vi "9-1.vi"() -> (3 "Numeric":i32)   [LabVIEW 2022 SP3, in "AoC22.lvlib"]
uses:
  AoC22.lvlib
  <vilib>/Utility/miscctls.llb/LVMapReplaceAction.ctl
  <vilib>/IlluminatedG/lv-stream/Stream.lvlib
panel:
  in  "OK Button":bool
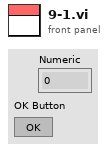
[diagram p1: front panel]
types:
  T1 = map{cluster{"Row":i32, "Col":i32}, cluster{"Tail Count":i32}}
  T2 = typedef "LVMapReplaceAction.ctl" = enum32{"Modify Entry only if found", "Add or Modify Entry", "Delete Entry"}
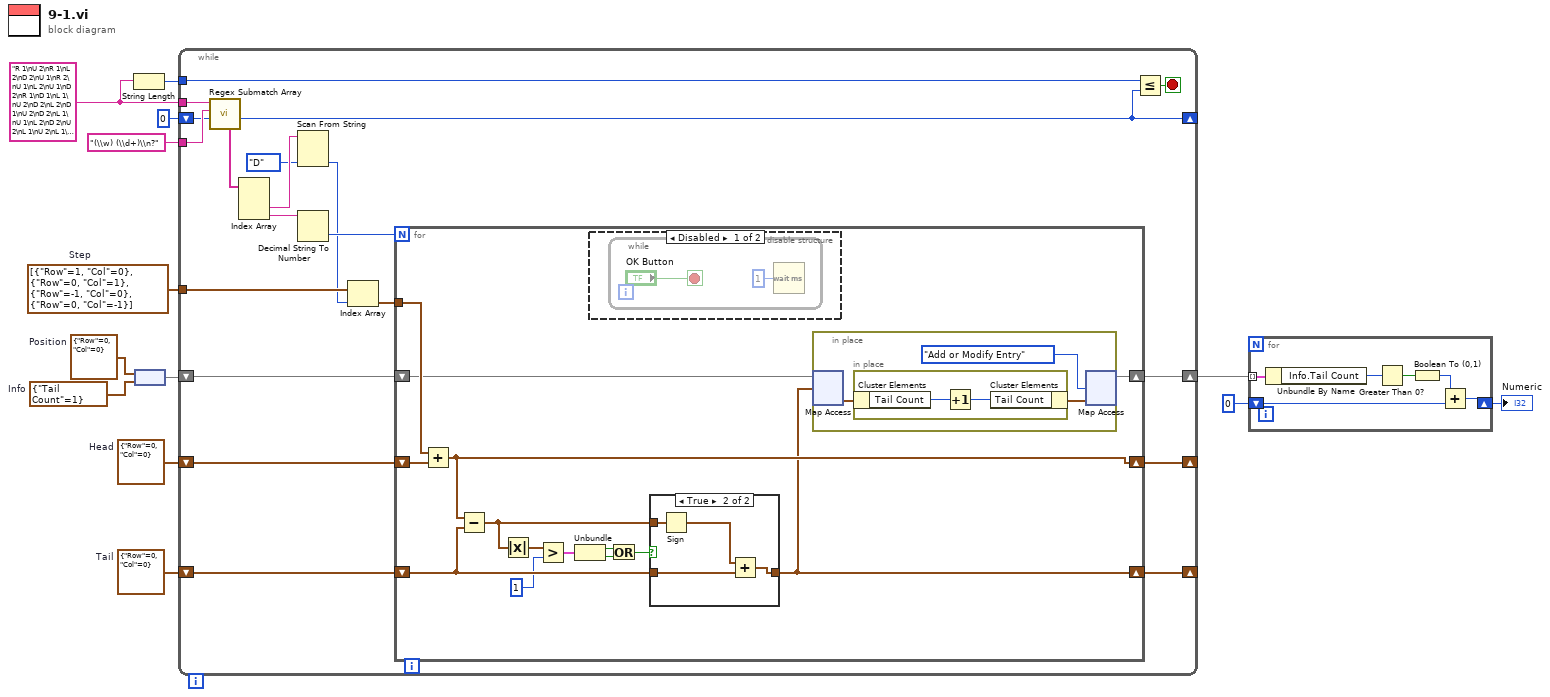
[diagram p0: block diagram]
diagram:
  w4 = cluster{"Tail Count":i32} {"Tail Count"=1}  # Info
  w6 = cluster{"Row":i32, "Col":i32} {"Row"=0, "Col"=0}  # Position
  w7 = cluster{"Row":i32, "Col":i32}[] [{"Row"=1, "Col"=0}, {"Row"=0, "Col"=1}, {"Row"=-1, "Col"=0}, {"Row"=0, "Col"=-1}]  # Step
  w11 = cluster{"Row":i32, "Col":i32} {"Row"=0, "Col"=0}  # Tail
  w12 = cluster{"Row":i32, "Col":i32} {"Row"=0, "Col"=0}  # Head
  w9 = "R 1\nU 2\nR 1\nL 2\nD 2\nU 1\nR 2\nU 1\nL 2\nU 1\nD 2\nR 1\nD 1\nL 1\nU 2\nD 2\nL 2\nD 1\nU 2\nD 2\nL 1\nU 1\nL 2\nD 2\nU 2\nL 1\nU 2\nL 1\nR 2\nU 1\nL 1\nR 2\nD 1\nU 2\nR 1\nU 1\nR 2\nU 1\nR 2\nU 1\nD 1\nU 1\nD 1\nL 2\nD 2\nR 1\nU 1\nR 1\nU 1\nL 1\nU 1\nD 2\nR 2\nD 2\nL 2\nU 2\nR 1\nD 1\nU 1\nD 2\nR 1\nD 2\nL 2\nR 2\nL 1\nU 1\nL 2\nD 2\nL 2\nD 1\nR 1\nL 2\nD 2\nR 1\nL 1\nR 1\nD 1\nR 1\nD 2\nL 2\nU 1\nD 2\nR 2\nD 1\nU 1\nL 1\nD 1\nU 2\nR 1\nU 1\nL 2\nU 1\nL 1\nU 2\nL 2\nD 2\nU 1\nL 1\nU 2\nD 2\nL 2\nD 2\nR 2\nU 2\nL 2\nD 1\nU 1\nR 2\nD 2\nL 2\nR 2\nD 2\nL 1\nD 1\nU 2\nR 2\nD 3\nR 1\nU 3\nL 3\nD 2\nR 1\nD 1\nL 2\nD 1\nR 2\nU 3\nL 2\nU 2\nR 3\nU 3\nL 1\nD 3\nR 3\nU 2\nR 3\nU 3\nL 1\nD 3\nR 3\nL 2\nR 2\nL 3\nD 3\nR 2\nD 2\nR 2\nD 1\nR 1\nL 1\nD 2\nR 1\nD 2\nU 1\nR 2\nL 2\nR 2\nU 2\nR 2\nD 1\nU 1\nD 1\nL 3\nU 3\nD 3\nL 1\nU 2\nR 2\nU 2\nR 1\nU 1\nL 2\nU 2\nR 3\nU 1\nD 3\nR 3\nU 2\nR 1\nU 1\nD 3\nL 2\nU 3\nL 1\nR 2\nD 3\nR 2\nU 1\nR 2\nD 1\nU 3\nL 2\nD 1\nR 1\nL 3\nR 3\nD 2\nR 1\nU 2\nR 3\nD 2\nU 2\nL 2\nU 1\nR 2\nU 2\nL 2\nD 3\nL 2\nD 1\nL 1\nU 2\nL 1\nD 2\nR 1\nD 2\nR 1\nL 2\nU 1\nL 1\nU 1\nD 2\nR 4\nD 4\nL 2\nR 4\nD 1\nL 2\nD 2\nL 4\nU 4\nD 4\nL 3\nR 3\nD 1\nL 1\nD 1\nU 4\nR 4\nU 4\nD 2\nR 1\nU 3\nR 2\nU 3\nR 4\nD 3\nU 3\nL 4\nD 1\nR 2\nU 3\nD 4\nU 3\nR 2\nL 1\nD 2\nU 2\nR 3\nU 2\nR 2\nD 2\nL 2\nU 4\nR 1\nL 3\nR 1\nL 1\nD 3\nR 4\nD 2\nR 4\nU 3\nL 1\nD 1\nR 4\nU 3\nD 1\nL 3\nR 1\nL 3\nD 2\nL 2\nR 3\nL 4\nD 4\nU 1\nL 1\nR 1\nD 3\nL 2\nR 1\nD 3\nR 2\nD 4\nU 4\nR 3\nU 1\nD 3\nL 3\nD 3\nU 1\nD 2\nU 4\nR 4\nU 2\nD 1\nR 1\nD 4\nL 2\nR 3\nU 4\nL 1\nD 1\nU 4\nL 3\nD 4\nU 2\nR 4\nU 2\nR 4\nU 2\nL 1\nR 1\nL 3\nD 4\nL 2\nR 2\nL 3\nU 3\nR 4\nL 2\nR 1\nD 5\nU 1\nR 1\nU 2\nR 1\nU 4\nL 3\nU 4\nR 2\nD 3\nL 4\nR 3\nL 2\nU 2\nR 1\nL 3\nD 5\nR 3\nL 2\nU 5\nR 2\nU 5\nL 5\nU 4\nR 4\nD 2\nR 4\nD 3\nR 2\nD 3\nU 2\nL 3\nD 3\nL 1\nU 4\nD 3\nL 1\nD 1\nR 2\nL 4\nR 3\nU 1\nR 3\nL 2\nR 3\nD 4\nR 2\nU 3\nL 4\nR 5\nL 1\nU 1\nD 5\nU 2\nR 5\nL 4\nD 3\nL 1\nD 3\nU 1\nR 2\nD 1\nL 5\nD 2\nR 4\nL 1\nD 2\nR 4\nL 3\nR 3\nL 3\nR 4\nL 3\nU 3\nD 4\nU 2\nR 1\nD 1\nU 1\nR 5\nD 5\nL 5\nR 3\nU 2\nD 4\nL 5\nD 1\nL 4\nR 4\nU 2\nL 2\nR 2\nU 3\nL 1\nU 3\nL 1\nD 4\nU 5\nD 5\nR 4\nL 4\nR 5\nD 4\nU 5\nL 4\nU 1\nD 4\nR 5\nD 2\nU 4\nR 2\nU 3\nD 2\nU 6\nD 4\nR 1\nD 4\nR 3\nL 1\nR 5\nU 6\nD 5\nL 4\nR 3\nL 4\nR 5\nD 1\nR 3\nD 2\nL 6\nU 5\nR 6\nL 2\nD 6\nU 1\nL 3\nD 4\nR 6\nD 3\nL 3\nR 5\nU 6\nD 5\nU 1\nR 4\nL 4\nU 4\nR 5\nD 1\nL 4\nU 6\nL 2\nR 3\nL 2\nR 3\nL 3\nR 4\nU 3\nD 1\nR 6\nD 5\nL 2\nR 4\nU 4\nD 2\nL 1\nR 2\nD 3\nL 4\nD 4\nR 4\nD 6\nR 1\nL 2\nR 5\nD 3\nU 5\nR 4\nL 6\nD 6\nU 4\nR 4\nL 4\nU 4\nR 5\nD 1\nU 1\nR 4\nL 2\nU 6\nD 3\nL 3\nU 6\nD 1\nU 4\nD 6\nR 6\nU 1\nR 2\nU 5\nD 4\nL 2\nU 5\nD 1\nL 5\nU 1\nR 3\nD 2\nR 1\nL 3\nD 1\nR 1\nL 2\nR 6\nD 6\nR 4\nU 4\nL 5\nR 6\nL 5\nR 4\nD 3\nL 2\nR 4\nL 2\nU 6\nD 5\nR 1\nL 3\nR 1\nU 2\nR 6\nL 2\nD 7\nL 2\nD 4\nR 2\nU 6\nD 4\nR 5\nU 6\nR 3\nL 3\nU 2\nR 3\nU 1\nR 7\nU 2\nR 2\nD 7\nR 1\nU 5\nD 1\nL 5\nU 5\nR 2\nD 5\nR 4\nU 5\nL 3\nD 4\nL 6\nR 7\nL 2\nD 3\nL 2\nD 6\nU 6\nL 1\nD 7\nU 6\nL 7\nR 5\nL 1\nU 7\nR 1\nL 4\nR 4\nL 5\nU 7\nD 4\nR 7\nL 5\nU 7\nL 6\nU 3\nD 5\nR 5\nU 7\nR 5\nL 3\nU 6\nR 2\nU 3\nR 3\nU 6\nL 5\nD 6\nL 4\nD 5\nR 1\nL 3\nU 6\nR 6\nU 6\nL 1\nD 2\nL 5\nD 1\nL 6\nU 5\nD 5\nR 5\nD 6\nL 4\nU 5\nR 2\nU 4\nD 7\nL 1\nU 1\nD 1\nL 1\nD 4\nU 1\nL 6\nU 1\nR 5\nD 1\nU 1\nR 1\nU 5\nR 4\nU 5\nL 2\nU 6\nL 7\nR 2\nU 4\nR 5\nL 1\nR 8\nL 2\nD 7\nR 7\nD 2\nL 2\nR 2\nD 2\nU 7\nD 7\nR 4\nU 1\nR 2\nL 6\nU 1\nL 3\nU 2\nD 7\nR 6\nL 5\nD 1\nL 3\nU 6\nD 2\nU 2\nR 4\nD 1\nL 7\nU 3\nD 8\nU 4\nD 8\nL 8\nU 6\nL 3\nU 4\nR 4\nU 8\nD 1\nR 7\nU 5\nL 8\nU 4\nL 4\nD 7\nU 8\nL 2\nD 8\nL 1\nR 1\nL 1\nR 8\nL 8\nR 5\nL 1\nR 4\nD 3\nR 2\nU 8\nL 6\nR 4\nL 3\nR 8\nL 4\nD 5\nR 3\nU 2\nD 8\nU 4\nR 6\nD 4\nR 3\nL 7\nD 8\nL 2\nU 6\nD 7\nR 3\nL 5\nR 4\nD 3\nL 4\nR 8\nL 7\nD 8\nR 3\nU 3\nL 3\nR 6\nL 1\nU 3\nL 1\nU 4\nR 8\nL 8\nR 2\nD 3\nL 2\nR 1\nD 2\nR 6\nU 3\nD 1\nU 3\nR 1\nU 2\nR 2\nL 2\nD 6\nU 7\nL 8\nD 6\nU 2\nR 3\nL 6\nU 9\nD 6\nU 1\nD 3\nU 4\nR 3\nL 9\nD 6\nU 9\nD 1\nL 5\nU 5\nD 6\nU 4\nL 8\nU 8\nD 3\nL 3\nU 9\nR 5\nL 7\nD 1\nR 9\nU 8\nD 1\nR 1\nU 9\nD 4\nR 6\nU 8\nR 6\nU 3\nD 2\nU 8\nL 8\nU 9\nD 4\nL 3\nU 4\nD 3\nL 9\nR 7\nL 9\nR 3\nL 5\nD 7\nL 8\nU 9\nL 7\nD 1\nL 6\nU 7\nL 6\nD 8\nU 9\nL 7\nR 7\nD 1\nR 6\nD 4\nU 7\nR 7\nL 8\nD 4\nR 1\nL 7\nD 2\nU 3\nD 1\nR 7\nD 7\nR 7\nL 6\nD 9\nU 7\nD 5\nR 7\nL 1\nR 9\nU 1\nL 2\nU 5\nR 4\nD 7\nR 2\nD 5\nU 4\nD 3\nR 9\nU 2\nD 9\nU 1\nR 9\nU 9\nD 1\nL 7\nU 6\nD 6\nU 9\nL 5\nU 2\nD 6\nL 4\nD 3\nU 1\nR 2\nL 1\nR 1\nD 1\nR 1\nU 1\nR 4\nL 7\nR 2\nD 1\nU 3\nD 3\nR 10\nL 7\nR 7\nD 2\nL 6\nR 9\nU 9\nD 8\nU 9\nR 2\nU 6\nD 9\nU 1\nL 2\nR 10\nL 9\nR 10\nL 6\nR 4\nD 4\nR 4\nU 4\nD 4\nL 5\nR 8\nD 4\nL 7\nD 6\nL 8\nR 9\nL 8\nD 7\nR 2\nU 2\nD 5\nL 4\nR 8\nD 7\nR 6\nD 7\nL 5\nU 7\nR 1\nD 7\nR 9\nD 5\nU 3\nL 8\nD 7\nU 4\nD 4\nR 10\nU 7\nD 4\nU 2\nR 7\nL 4\nU 2\nD 9\nL 5\nR 2\nU 10\nL 9\nR 10\nL 1\nD 5\nR 10\nL 5\nR 5\nD 5\nR 10\nL 4\nU 9\nD 7\nR 10\nL 6\nU 3\nD 5\nU 6\nL 6\nU 10\nL 1\nU 10\nD 4\nL 7\nU 2\nL 10\nR 4\nL 7\nR 4\nD 10\nL 4\nU 10\nL 10\nD 9\nU 4\nR 8\nU 8\nR 5\nU 3\nD 10\nR 7\nL 10\nR 9\nL 1\nD 6\nL 11\nD 11\nR 3\nL 8\nU 6\nR 9\nD 5\nR 9\nD 4\nU 7\nD 4\nR 4\nU 10\nD 4\nR 2\nL 3\nU 5\nD 11\nR 8\nL 8\nU 7\nR 3\nD 8\nU 5\nR 10\nD 5\nR 2\nU 11\nD 10\nR 1\nU 9\nL 10\nR 2\nD 11\nR 6\nL 3\nR 10\nU 2\nD 6\nL 10\nU 5\nL 6\nU 1\nR 10\nU 8\nR 8\nD 4\nU 8\nL 11\nR 7\nL 2\nD 2\nR 5\nU 10\nL 3\nR 6\nL 8\nR 8\nU 8\nD 3\nL 7\nR 5\nL 6\nD 11\nL 6\nD 7\nU 6\nD 3\nU 9\nL 7\nR 8\nL 3\nR 10\nD 11\nL 11\nR 4\nD 6\nL 7\nD 9\nR 10\nU 11\nL 9\nD 8\nL 2\nU 1\nD 7\nU 10\nD 11\nR 5\nD 11\nL 6\nD 5\nR 6\nD 5\nR 11\nU 3\nD 6\nR 5\nU 7\nD 2\nR 6\nU 5\nD 9\nU 3\nR 7\nD 10\nU 5\nD 4\nR 6\nU 11\nL 10\nU 5\nL 6\nR 5\nU 7\nL 7\nR 5\nD 9\nU 11\nL 7\nU 8\nL 7\nU 3\nL 8\nR 10\nU 11\nR 8\nL 12\nU 8\nD 2\nL 2\nD 2\nU 10\nR 11\nU 2\nR 6\nU 3\nD 9\nU 5\nD 12\nL 11\nD 8\nU 12\nR 4\nU 1\nL 2\nR 10\nD 6\nL 10\nU 2\nR 4\nL 4\nD 8\nU 9\nL 4\nD 10\nU 5\nR 10\nL 2\nD 2\nU 2\nR 7\nD 8\nR 1\nU 11\nD 1\nL 7\nR 12\nD 12\nR 3\nL 11\nR 10\nU 11\nR 5\nD 6\nR 11\nD 2\nL 3\nD 12\nL 9\nR 6\nU 1\nD 2\nR 6\nD 5\nU 7\nR 2\nD 5\nU 3\nD 12\nR 12\nL 9\nR 9\nD 12\nR 8\nD 11\nL 7\nU 4\nD 11\nR 1\nU 9\nL 1\nD 2\nR 3\nU 1\nD 1\nR 2\nD 11\nU 12\nR 7\nD 1\nU 13\nL 5\nD 13\nL 10\nD 12\nL 7\nD 9\nL 7\nU 6\nL 1\nR 1\nL 10\nR 7\nL 6\nU 7\nR 10\nU 7\nR 11\nU 12\nL 2\nD 11\nL 5\nU 2\nD 8\nL 10\nD 13\nU 10\nL 9\nU 5\nD 11\nR 6\nL 9\nR 2\nL 6\nU 4\nR 7\nD 11\nL 3\nU 6\nD 13\nU 2\nR 13\nU 11\nL 12\nD 13\nL 1\nR 9\nD 10\nU 6\nL 13\nU 2\nL 12\nD 7\nR 1\nL 6\nD 1\nU 10\nD 5\nL 2\nU 12\nR 1\nU 9\nD 4\nU 10\nL 1\nR 1\nU 8\nR 2\nD 1\nL 6\nU 11\nD 2\nU 7\nD 11\nU 9\nD 6\nU 5\nD 13\nR 2\nU 8\nL 4\nU 4\nR 2\nU 1\nD 3\nL 1\nD 13\nR 9\nL 4\nD 5\nL 7\nU 2\nD 10\nL 6\nU 11\nD 1\nU 5\nR 4\nD 9\nR 12\nD 2\nU 9\nL 10\nU 6\nD 2\nL 8\nU 4\nL 4\nD 12\nU 3\nL 14\nD 12\nR 12\nL 7\nU 5\nL 2\nD 4\nL 13\nD 10\nL 8\nD 12\nR 13\nU 8\nD 14\nU 4\nR 11\nL 4\nR 13\nL 2\nU 1\nD 10\nL 12\nD 13\nL 4\nD 11\nR 14\nU 8\nL 11\nD 2\nU 8\nL 8\nD 3\nL 14\nU 7\nL 2\nR 2\nD 6\nU 1\nL 12\nR 12\nU 4\nL 1\nU 13\nR 12\nD 8\nU 10\nR 2\nL 7\nR 4\nD 4\nL 14\nU 2\nD 2\nU 11\nL 7\nR 12\nU 9\nL 11\nR 6\nD 6\nR 8\nL 1\nD 9\nL 7\nD 10\nR 6\nD 6\nL 5\nD 14\nL 12\nU 12\nR 4\nD 14\nL 10\nD 11\nL 3\nD 3\nU 9\nL 6\nD 10\nU 1\nL 10\nD 9\nR 8\nL 3\nU 7\nR 4\nU 9\nL 5\nR 7\nD 7\nL 5\nU 4\nR 4\nL 7\nR 8\nL 2\nR 5\nL 10\nR 2\nL 12\nD 12\nL 6\nR 4\nL 11\nD 13\nL 13\nR 10\nD 12\nU 5\nR 11\nL 15\nR 6\nU 9\nD 5\nU 6\nL 1\nD 1\nR 7\nD 5\nR 15\nU 11\nR 5\nD 15\nR 13\nU 8\nR 11\nU 7\nD 4\nL 6\nD 11\nU 1\nL 2\nR 11\nL 12\nD 5\nR 3\nL 14\nR 15\nL 14\nU 13\nD 9\nL 3\nD 4\nU 9\nL 3\nR 14\nU 3\nR 15\nL 14\nR 4\nU 15\nL 1\nD 11\nL 13\nD 14\nL 1\nD 1\nU 13\nD 7\nU 13\nD 15\nU 15\nL 6\nD 7\nR 15\nL 10\nU 6\nR 7\nL 13\nU 3\nD 9\nL 3\nD 10\nR 14\nD 15\nL 6\nD 4\nU 11\nL 11\nD 6\nU 8\nD 15\nR 5\nL 9\nD 15\nU 15\nR 9\nD 11\nU 7\nL 9\nU 8\nD 2\nL 4\nD 11\nU 12\nR 11\nU 5\nL 12\nU 5\nR 14\nL 10\nR 6\nD 3\nL 13\nU 6\nR 10\nD 10\nU 9\nD 3\nR 7\nL 13\nR 15\nU 6\nL 13\nU 11\nD 9\nL 7\nR 8\nU 6\nR 12\nU 2\nL 8\nU 10\nD 11\nU 14\nR 3\nL 15\nU 9\nL 2\nU 2\nD 11\nL 11\nR 3\nD 14\nU 3\nL 1\nU 2\nD 12\nL 5\nR 5\nD 10\nL 16\nR 4\nU 3\nL 6\nR 9\nL 7\nR 2\nU 15\nR 6\nL 12\nD 16\nL 16\nD 15\nU 12\nL 6\nD 9\nU 8\nL 10\nD 11\nU 4\nD 12\nU 7\nD 14\nU 1\nD 10\nR 10\nD 14\nL 5\nD 6\nR 8\nL 16\nU 7\nL 12\nR 13\nL 11\nD 12\nR 5\nD 11\nL 5\nR 4\nD 15\nL 13\nD 10\nR 2\nL 16\nD 14\nR 15\nD 11\nU 2\nD 12\nL 11\nD 1\nR 5\nD 6\nU 13\nL 10\nR 1\nU 10\nD 12\nL 10\nD 10\nR 11\nL 10\nD 11\nL 3\nR 11\nD 12\nL 6\nU 2\nL 10\nD 9\nL 11\nU 12\nD 14\nL 6\nU 16\nD 2\nL 2\nD 14\nU 7\nR 12\nD 14\nL 4\nU 3\nR 16\nD 2\nL 5\nR 10\nL 1\nR 11\nL 14\nD 3\nL 17\nD 4\nU 1\nR 8\nD 8\nL 5\nU 1\nL 13\nD 15\nU 17\nL 1\nD 14\nU 4\nR 1\nU 2\nD 14\nR 10\nU 14\nD 17\nR 10\nU 13\nD 12\nU 8\nL 11\nU 17\nR 12\nU 6\nD 8\nR 10\nU 16\nD 4\nR 3\nD 3\nU 4\nL 3\nU 5\nR 16\nL 5\nR 16\nD 17\nR 12\nL 11\nR 13\nU 12\nL 8\nR 5\nD 6\nU 16\nL 16\nD 2\nL 11\nD 1\nR 1\nD 14\nR 15\nL 6\nU 14\nR 12\nD 11\nL 9\nU 6\nL 11\nD 15\nU 17\nL 1\nU 3\nL 6\nU 5\nR 16\nL 14\nR 9\nL 12\nD 14\nU 13\nL 3\nU 13\nD 7\nR 2\nU 7\nD 5\nL 17\nD 6\nL 16\nR 5\nD 4\nR 3\nU 11\nD 3\nU 9\nD 10\nU 2\nL 6\nD 6\nR 15\nD 17\nR 1\nL 15\nD 2\nU 5\nR 2\nD 6\nL 8\nR 5\nL 2\nD 17\nU 9\nD 9\nL 7\nR 12\nL 12\nR 18\nL 10\nR 9\nD 6\nR 9\nU 15\nL 17\nD 18\nR 1\nL 15\nD 4\nR 6\nU 3\nR 6\nU 3\nD 1\nU 9\nD 8\nR 3\nD 6\nU 3\nR 8\nL 8\nR 10\nU 7\nD 16\nU 17\nR 11\nU 8\nD 1\nU 8\nL 4\nR 12\nD 10\nU 7\nD 18\nU 7\nD 12\nL 18\nU 9\nR 2\nU 5\nD 14\nR 13\nD 15\nU 17\nD 16\nL 4\nD 10\nL 2\nU 7\nL 7\nD 13\nR 13\nU 12\nR 16\nU 17\nR 3\nU 12\nR 6\nD 12\nU 11\nL 6\nU 15\nL 12\nR 1\nD 6\nL 16\nR 1\nD 7\nR 17\nL 15\nD 15\nU 9\nR 18\nD 13\nR 14\nD 1\nR 1\nD 16\nL 18\nR 1\nU 14\nL 8\nD 14\nR 15\nD 2\nU 10\nD 17\nU 3\nD 9\nR 7\nD 17\nU 3\nD 15\nL 17\nD 17\nR 1\nD 10\nL 9\nD 14\nR 5\nU 14\nR 14\nD 12\nR 18\nU 4\nD 2\nU 17\nD 12\nL 4\nU 9\nL 9\nU 17\nR 4\nU 17\nR 8\nD 10\nR 3\nD 9\nU 17\nL 5\nR 16\nU 9\nL 5\nD 15\nU 2\nD 7\nL 15\nU 1\nL 16\nR 8\nL 13\nR 3\nD 8\nR 1\nD 8\nL 10\nU 16\nR 16\nL 2\nU 3\nD 9\nU 12\nD 1\nL 10\nD 15\nU 7\nR 3\nD 15\nU 4\nL 6\nR 14\nU 13\nR 16\nU 2\nR 9\nU 15\nD 8\nL 8\nR 17\nD 3\nL 17\nD 13\nU 8\nD 11\nR 13\nL 3\nD 2\nU 14\nR 1\nU 10\nR 11\nD 16\nL 10\nR 17\nU 7\nL 13\nR 3\nL 18\nR 5\nU 7\nL 12\nD 4\nU 5\nL 17\nR 18\nL 4\nR 19\nL 12\nU 17\nR 2\nL 11\nR 9\nD 16\nR 19\nL 18\nU 11\nD 4\nR 13\nL 18\nU 13\nR 19\nD 3\nR 10\nL 3\nR 5\nD 2\nR 2\nL 18\nD 15\nR 19\nL 5\nD 4\nU 5\nR 12\nD 15\nL 13\nR 16\nU 16\nL 6\nU 12\nL 8"
  n1 = String Length(string=w9) -> (length=w8:i32)
  n2 = node(w6, w4) -> (w5:T1)
  n3 = while {
    tunnel: w9 -> [w33]
    tunnel: "(\\w) (\\d+)\\n?" ("regular expression") -> [w28]
    shift-right: [w15] -> _
    shift-left: w12 -> [w19]
    shift-right: [w14] -> _
    shift-left: w11 -> [w18]
    shift-right: [w25] -> _
    shift-left: 0 ("offset past match") -> [w27]
    tunnel: w8 -> [w26]
    shift-right: [w16] -> w3
    shift-left: w5 -> [w17]
    tunnel: w7 -> [w22]
    stop <- w24 stop-if-true
    n4 = call <vilib>:"Regex Submatch Array.vi"("offset (0)"=w27, "regular expression"=w28, "string"=w33) -> ("offset past match"=w25:i32, "matches"=w32:string[])  [unwired: 6 in, 1 out]
    n5 = Index Array(array=w32) -> (element #2=w30:string, element #3=w31:string)  [unwired: 3 in, 1 out]
    n6 = Scan From String(input string=w30, default 1=enum16{"U", "R", "D", "L"}."D") -> (output 1=w21:enum16{"U", "R", "D", "L"})  [unwired: 3 in, 3 out]
    n7 = Decimal String To Number(string=w31) -> (number=w23:i32)  [unwired: 2 in, 1 out]
    n8 = Index Array(array=w22, index=w21) -> (element=w20:cluster{"Row":i32, "Col":i32})
    n9 = for {
      N: w23 -> [_]
      shift-right: [w45] -> w15
      shift-left: w19 -> [w47]
      shift-right: [w42] -> w14
      shift-left: w18 -> [w44]
      tunnel: w20 -> [w46]
      shift-right: [w41] -> w16
      shift-left: w17 -> [w34]
      n10 = Add(x=w46, y=w47) -> (x+y=w45:cluster{"Row":i32, "Col":i32})
      n11 = Subtract(x=w45, y=w44) -> (x-y=w43:cluster{"Row":i32, "Col":i32})
      n12 = Absolute Value(x=w43) -> (abs(x)=w40:cluster{"Row":i32, "Col":i32})
      n13 = Greater?(x=w40, y=1) -> (0:w36:cluster{"Row":bool, "Col":bool})
      n14 = Unbundle(w36) -> ("Row"=w37:bool, "Col"=w38:bool)
      n15 = disable-structure shown="Disabled" {
        frame Disabled {
          n16 = while {
            stop <- "OK Button" stop-if-true
            n17 = Wait (ms)(milliseconds to wait=u32 1) -> ()  [unwired: 1 out]
          }
        }
        frame Enabled {
        }
      }
      n18 = Or(x=w37, y=w38) -> (x .or. y?=w35:bool)
      n19 = case shown="True" w35 {
        tunnel: w44 -> [w50 w53]
        tunnel: w43 -> [_ w54]
        tunnel: [w50 w51] -> w42
        frame False {
        }
        frame True {
          n20 = Sign(1:w54) -> (0:w52:cluster{"Row":i32, "Col":i32})
          n21 = Add(x=w52, y=w53) -> (x+y=w51:cluster{"Row":i32, "Col":i32})
        }
      }
      n22 = in-place {
        n23 = in-place-map #1(w34, w42) -> (w56:cluster{"Tail Count":i32})  [unwired: 1 in, 1 out]
        n24 = in-place {
          n25 = in-place-cluster #2(w56) -> ("Tail Count"=w59:i32)
          n26 = Increment(x=w59) -> (x+1=w58:i32)
          n27 = in-place-cluster #2("Tail Count"=w58) -> (w55:cluster{"Tail Count":i32})
        }
        n28 = in-place-map #1(w55, LVMapReplaceAction."Add or Modify Entry" ("action")) -> (w41:T1)  [unwired: 2 out]
      }
    }
    n29 = Less Or Equal?(x=w26, y=w25) -> (x <= y?=w24:bool)
  }
  n30 = for {
    tunnel: w3 -> [w65] mode=indexing
    shift-right: [w60] -> w1
    shift-left: 0 -> [w61]
    n31 = Unbundle By Name(w65) -> ("Info.Tail Count"=w64:i32)
    n32 = Greater Than 0?(x=w64) -> (x > 0?=w63:bool)
    n33 = Boolean To (0,1)(Boolean=w63) -> (0, 1=w62:i16)
    n34 = Add(x=w62, y=w61) -> (x+y=w60:i32)
  }
  "Numeric" <- w1
